vi "Omni wheel output.vi"(6 "input angle":dbl, 8 "error in":errorcluster, 11 "motor angle":dbl) -> (0 "error out":errorcluster, 3 "speed multiplier":dbl format="%#.4f")   [LabVIEW 2017]
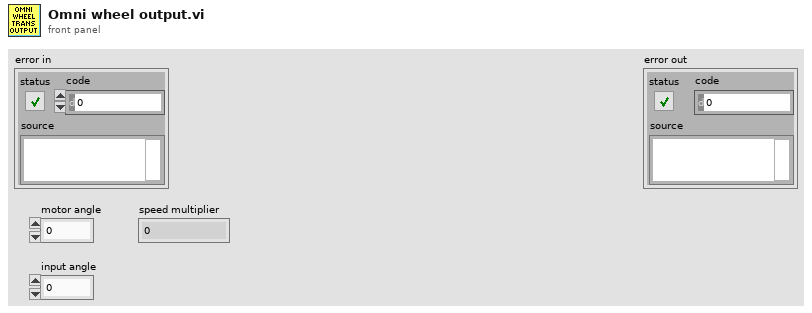
[diagram p1: front panel]
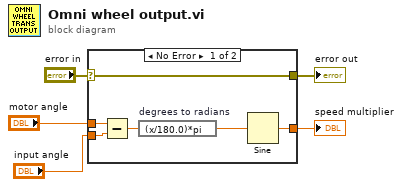
[diagram p0: block diagram]
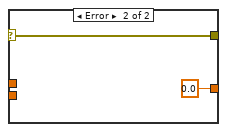
[diagram p2: hidden frame]
diagram:
  n1 = case shown="No Error" "error in" {
    selector: "error in" -> [w6 w12]
    tunnel: [w11 0.0] -> w5
    tunnel: "input angle" -> [w8 _]
    tunnel: "motor angle" -> [w7 _]
    tunnel: [w6 w12] -> w2
    frame No Error {
      n2 = Subtract(x=w7, y=w8) -> (x-y=w9:dbl)
      n3 = expression code="(x/180.0)*pi" "degrees to radians"(w9) -> (w10:dbl)
      n4 = Sine(x=w10) -> (sin(x)=w11:dbl)
    }
    frame Error {
    }
  }
  "speed multiplier" <- w5
  "error out" <- w2
